vi "SOAE-End Acquisition.vi"(0 "runtime":T1, 11 "error in (no error)":errorcluster) -> (15 "error out":errorcluster)   [LabVIEW 2020]
uses:
  Typedefs/SOAE-Acq Runtime.ctl
  Utility VIs/Math VIs/Linear to dB (array).vi
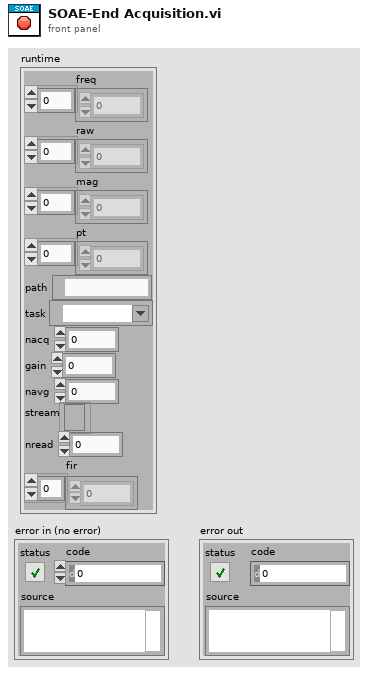
[diagram p1: front panel]
types:
  T1 = typedef "SOAE-Acq Runtime.ctl" = cluster{"freq":dbl[], "raw":dbl[], "mag":dbl[], "pt":dbl[], "path":path, "task":refnum<k21>, "nacq":i32, "gain":dbl, "navg":i32, "stream":refnum<file>, "nread":i32, "fir":dbl[]}
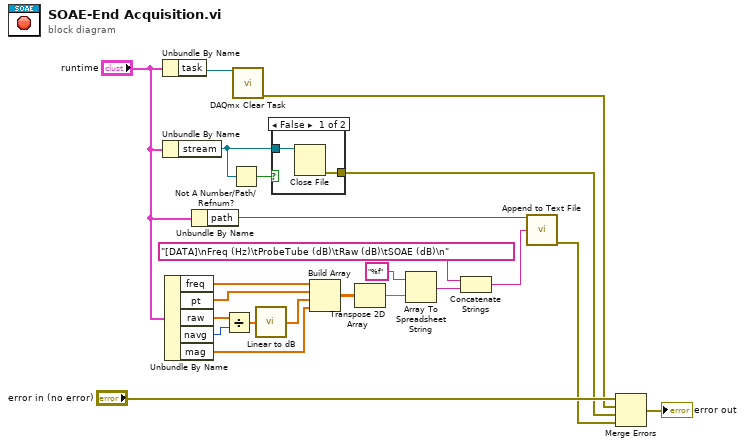
[diagram p0: block diagram]
diagram:
  n1 = Unbundle By Name("runtime") -> ("task"=w23:refnum<k21>)
  n2 = Unbundle By Name("runtime") -> ("stream"=w18:refnum<file>)
  n3 = Unbundle By Name("runtime") -> ("freq"=w16:dbl[], "pt"=w15:dbl[], "raw"=w14:dbl[], "navg"=w3:i32, "mag"=w1:dbl[])
  n4 = Unbundle By Name("runtime") -> ("path"=w8:path)
  n5 = Divide(x=w14, y=w3) -> (x/y=w4:dbl[])
  n6 = Not A Number/Path/Refnum?(number/path/refnum=w18) -> (NaN/Path/Refnum?=w19:bool)
  n7 = call <vilib>:"DAQmx Clear Task.vi"("task in"=w23) -> ("error out"=w20:errorcluster)  [unwired: 14 in]
  n8 = call-poly "Linear to dB.vi"("linear"=w4) -> ("dB"=w2:dbl[])
  n9 = case shown="False" w19 {
    tunnel: w18 -> [w25 _]
    tunnel: [w24 _] -> w17
    frame False {
      n10 = Close File(refnum=w25) -> (error out=w24:errorcluster)  [unwired: 1 in, 1 out]
    }
    frame True {
    }
  }
  n11 = Build Array(w16, w15, w2, w1) -> (w13:dbl[][])
  n12 = Transpose 2D Array(2D array=w13) -> (transposed array=w12:dbl[][])
  n13 = Array To Spreadsheet String(array=w12, 3:"%f" ("format string")) -> (spreadsheet string=w11:string)  [unwired: 1 in]
  n14 = Concatenate Strings("[DATA]\nFreq (Hz)\tProbeTube (dB)\tRaw (dB)\tSOAE (dB)\n", w11) -> (w7:string)
  n15 = call "Append to Text File.vi"("file path"=w8, "text"=w7) -> ("error out"=w6:errorcluster)  [unwired: 12 in, 1 out]
  n16 = Merge Errors("error in (no error)", w20, w17, w6) -> (→"error out":errorcluster)
